vi "ADIS16448_RoboRIO_Teensy_Close.vi"(8 "error in":errorcluster, 11 "SerialPortRef":T1) -> (0 "error out":errorcluster)   [LabVIEW 2016, in "RoboRIO-Teensy-ADIS16448-Interface.lvlib"]
uses:
  <vilib>/Rock Robotics/WPI/SerialPort/WPI_SerialPortRef.ctl
  RoboRIO-Teensy-ADIS16448-Interface.lvlib
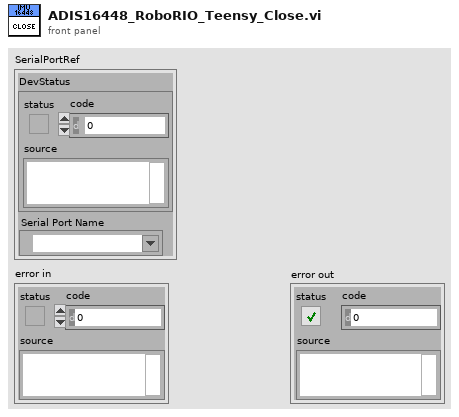
[diagram p1: front panel]
types:
  T1 = typedef "WPI_SerialPortRef.ctl" = cluster{"DevStatus":errorcluster, "Serial Port Name":refnum<visa-resource-name>}
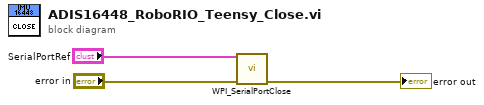
[diagram p0: block diagram]
diagram:
  n1 = call <vilib>:"WPI_SerialPortClose.vi"("error in (no error)"="error in", "SerialPortRef"="SerialPortRef") -> ("error out"=→"error out":errorcluster)  [unwired: 9 in]
